vi "UI Create.vi"(8 "error in (no error)":errorcluster, 10 "VI Refnum":refnum<vi>, 11 "GUI Control in":refnum<class "GUI Control.lvclass">) -> (0 "error out":errorcluster, 3 "GUI Control out":refnum<class "GUI Control.lvclass">)   [LabVIEW 2015, in "GUI Control.lvclass"]
uses:
  GUI Control.lvclass
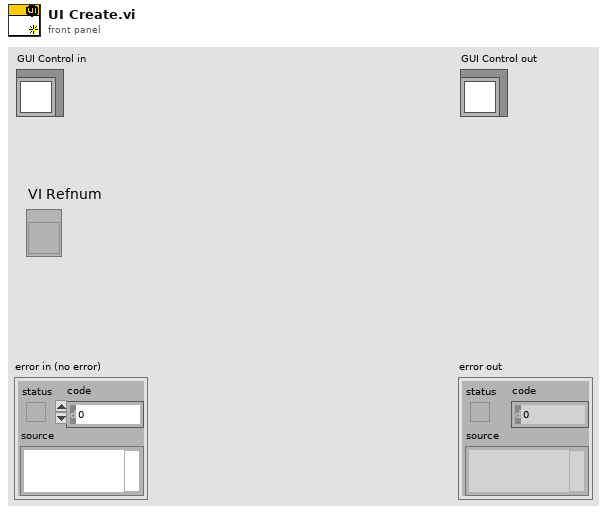
[diagram p1: front panel]
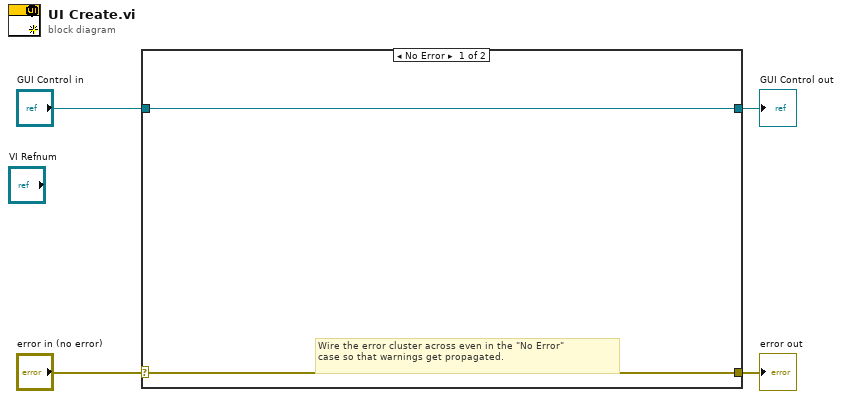
[diagram p0: block diagram]
diagram:
  n1 = case shown="No Error" "error in (no error)" {
    selector: "error in (no error)" -> [w5 w8]
    tunnel: [w5 w8] -> w3
    tunnel: [w6 w7] -> w1
    tunnel: "GUI Control in" -> [w6 w7]
    frame No Error {
      # "Wire the error cluster across even in the \"No Error\"\ncase so that warnings get propagated."
    }
    frame Error {
    }
  }
  "error out" <- w3
  "GUI Control out" <- w1
